vi "Read Config.vi"(8 "error in (no error)":errorcluster, 11 "PM_Group in":refnum<class "PM_Group.lvclass">) -> (0 "error out":errorcluster, 3 "PM_Group out":refnum<class "PM_Group.lvclass">)   [LabVIEW 2019, in "PM_Group.lvclass"]
uses:
  PM_Group.lvclass
  D:/GIT H4000/H4000/src/Device_class/Device.lvclass
  Device_class/Device.lvclass/Device.ctl
  PM_Group.lvclass/PM_Group.ctl
  SV_Puplisher_class/SV_Publisher.lvclass/SV_Publisher.ctl
  9c15e803-d321-4b59-aa33-b6832c2993ff.vi
  <vilib>/Utility/error.llb/Clear Errors.vi
  SV_Puplisher_class/Set SV.vi/1ae5d02c-efd0-450a-8aa4-8388e25d05bc.vi
  ConfigInterface_class/ConfigInterface.lvclass
  Device_class/Device.lvclass
  SV_Puplisher_class/SV_Publisher.lvclass
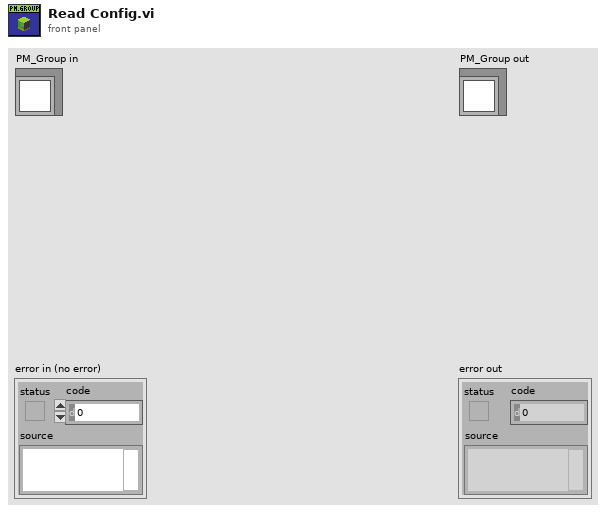
[diagram p1: front panel]
types:
  T1 = typedef "GUI Setting PMG.ctl" = cluster{"Temp Turn ON M24":dbl, "Temp Turn OFF M24":dbl, "Temp Open Water M21":dbl, "Temp Close Water M21":dbl, "H_51_on (cool)":dbl, "L_51_off (cool)":dbl, "H_52_off (oil)":dbl, "L_52_on (oil)":dbl}
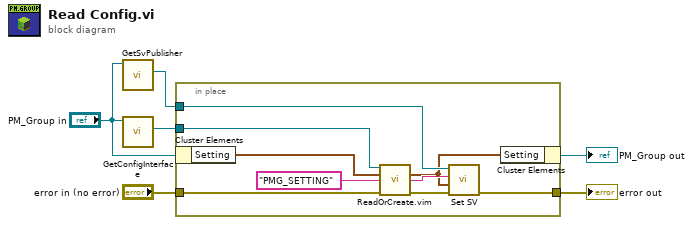
[diagram p0: block diagram]
diagram:
  n1 = call "GetSvPublisher.vi"("Device in"="PM_Group in") -> ("SV_Publisher.lvclass"=w1:refnum<class "SV_Publisher.lvclass">)  [unwired: 10 in]
  n2 = call "GetConfigInterface.vi"("Device in"="PM_Group in") -> ("ConfigInterface"=w6:refnum<class "ConfigInterface.lvclass">)  [unwired: 10 in]
  n3 = in-place {
    in-place-border: w6 -> [w15]
    in-place-border: "error in (no error)" -> [w12]
    in-place-border: [w7] -> w3
    in-place-border: w1 -> [w11]
    n4 = in-place-cluster #1("PM_Group in") -> ("Setting"=w13:T1)
    n5 = call "ReadOrCreate.vim"("reference in"=w15, "Type and Defaults"=w13, "Name"="PMG_SETTING", "error in (no error)"=w12) -> ("Data"=w9:T1, "Name dub"=w10:string, "error out"=w8:errorcluster)  [unwired: 7 in, 2 out]
    n6 = call "Set SV.vi"("error in (no error)"=w8, "SV Value"=w9, "SV Name"=w10, "SV_Publisher in"=w11) -> ("error out"=w7:errorcluster)  [unwired: 6 in, 1 out]
    n7 = in-place-cluster #1("Setting"=w9) -> (→"PM_Group out":refnum<class "PM_Group.lvclass">)
  }
  "error out" <- w3
